vi "subVI_read_ADC.vi"(11 "CH  2":bool[](array[boolean])=[FALSE, FALSE, TRUE, FALSE, FALSE, TRUE, FALSE, FALSE, FALSE, FALSE, FALSE, FALSE, FALSE, FALSE, FALSE, FALSE]) -> (0 "GAIN 2":i16, 1 "UNI 2":i16, 2 "FPGA VI Reference Out 2":refnum<k20>, 3 "error out 2":errorcluster, 4 "i 2":u32)   [LabVIEW 2018]
uses:
  <vilib>/Utility/error.llb/Error Cluster From Error Code.vi
  <vilib>/rvi/errors/niLvFpgaAdjustHostInterfaceError.vi
  <vilib>/rvi/interface/nirviReadWriteControl/nirviReadWriteControl.xnode
  NiFpgaLv.dll
  <vilib>/rvi/interface/Simulation/niFpgaSimulationCallBeginRW.vi
panel:
  in  "FPGA VI Reference In 2":refnum<k20>
  in  "error in 2":errorcluster
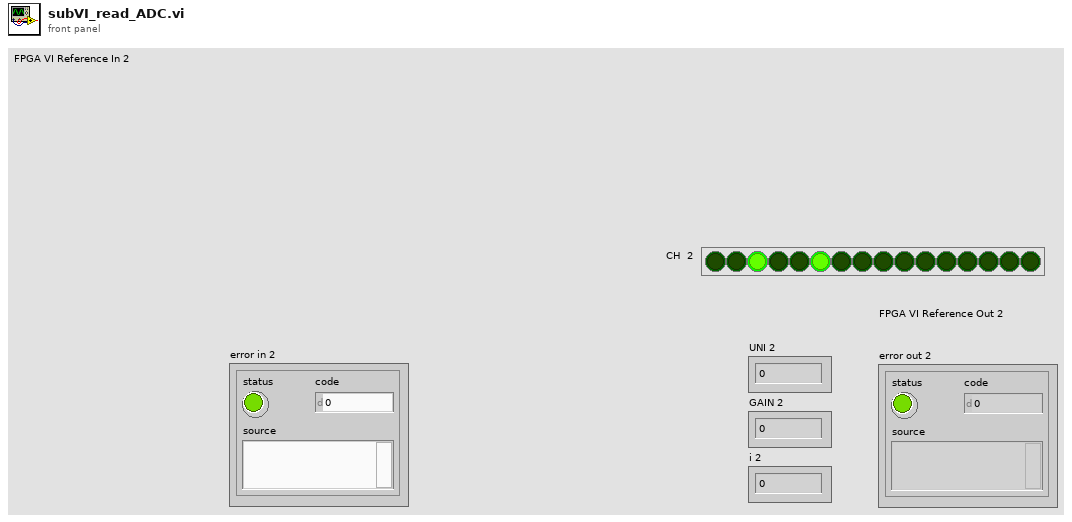
[diagram p1: front panel]
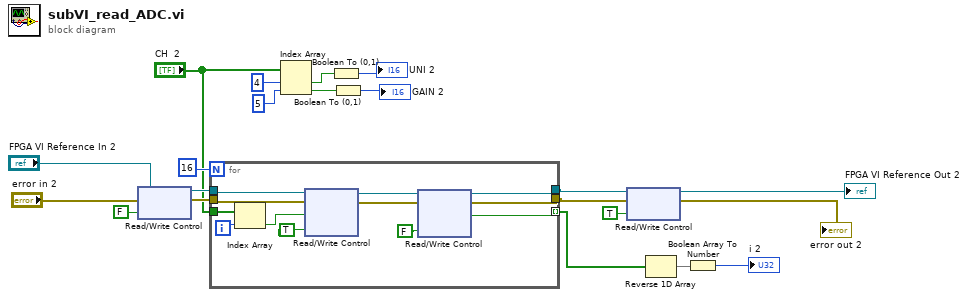
[diagram p0: block diagram]
diagram:
  n1 = xnode "Read/Write Control"("FPGA VI Reference In"="FPGA VI Reference In 2", "error in"="error in 2", "CS"=FALSE) -> ("FPGA VI Reference Out"=w13:refnum<k20>, "error out"=w12:errorcluster)
  n2 = for {
    N: 16 -> [_]
    tunnel: w13 -> [w30]
    tunnel: w12 -> [w29]
    tunnel: [w26] -> w3 mode=indexing
    tunnel: [w25] -> w15
    tunnel: [w24] -> w14
    tunnel: "CH  2" -> [w28]
    i -> [w27]
    n3 = Index Array(array=w28, index=w27) -> (element=w33:bool)
    n4 = xnode "Read/Write Control"("FPGA VI Reference In"=w30, "error in"=w29, "MOSI1"=w33, "CLK1"=TRUE ("CLK")) -> ("FPGA VI Reference Out"=w23:refnum<k20>, "error out"=w22:errorcluster)
    n5 = xnode "Read/Write Control"("FPGA VI Reference In"=w23, "error in"=w22, "CLK1"=FALSE ("CLK2")) -> ("FPGA VI Reference Out"=w25:refnum<k20>, "error out"=w24:errorcluster, "MISO1"=w26:bool)
  }
  n6 = Index Array(array="CH  2", index #1=4 ("index"), index #2=5 ("index")) -> (element #1=w17:bool, element #2=w16:bool)
  n7 = Boolean To (0,1)(Boolean=w17) -> (0, 1=→"UNI 2":i16)
  n8 = Boolean To (0,1)(Boolean=w16) -> (0, 1=→"GAIN 2":i16)
  n9 = xnode "Read/Write Control"("FPGA VI Reference In"=w15, "error in"=w14, "CS"=TRUE) -> ("FPGA VI Reference Out"=→"FPGA VI Reference Out 2":refnum<k20>, "error out"=→"error out 2":errorcluster)
  n10 = Reverse 1D Array(array=w3) -> (reversed array=w2:bool[])
  n11 = Boolean Array To Number(Boolean array=w2) -> (number=→"i 2":u32)
